vi "Mutate Status Glyph.vi"(8 "error in":errorcluster, 11 "device in":T1 format="%.0x") -> (0 "error out":errorcluster, 3 "device out":T1 format="%.0x")   [LabVIEW 2027, in "Embedded Data Logger System Explorer.lvlib"]
uses:
  Embedded Data Logger System Explorer.lvlib
  <vilib>/NI VeriStand/Custom Device API/Custom Device Item Ref.ctl
  Shared/Constants.vi
  <vilib>/NI VeriStand/Custom Device Tools/Custom Device Utility Library/NI VeriStand - Search for All Items by GUID.vi
  <vilib>/NI VeriStand/Custom Device Tools/Custom Device Utility Library/Custom Device Utility Library.lvlib
  Shared/Embedded Data Logger Shared.lvlib
  <vilib>/NI VeriStand/Custom Device API/Custom Device API.lvlib
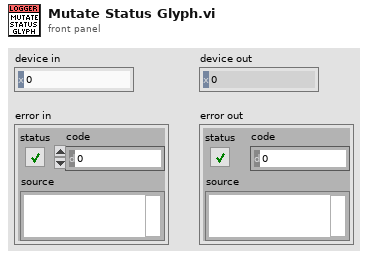
[diagram p1: front panel]
types:
  T1 = typedef "Custom Device API.lvlib/Custom Device Item Ref.ctl" = u64
  T2 = typedef "Custom Device API.lvlib/Custom Device Item Info.ctl" = cluster{"Name":string, "Is Channel":bool, "GUID":string, "Is Waveform":bool}
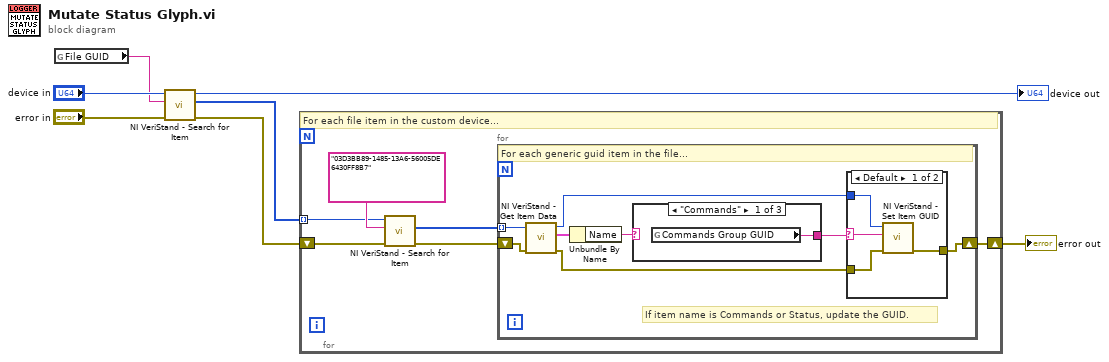
[diagram p0: block diagram]
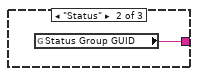
[diagram p3: hidden frame]
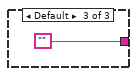
[diagram p4: hidden frame]
diagram:
  n1 = global read "Constants.vi" "File GUID"() -> (w2:string)
  n2 = call-poly <vilib>:"NI VeriStand - Search for Item.vi"("error in"="error in", "Item GUID"=w2, "Section Ref in"="device in") -> ("error out"=w6:errorcluster, "Item Refs"=w7:T1[], "Section Ref out"=→"device out":T1)  [unwired: 1 in, 5 out]
  n3 = for {
    shift-right: [w8] -> w1
    shift-left: w6 -> [w10]
    tunnel: w7 -> [w12] mode=indexing
    # "For each file item in the custom device..."
    n4 = call-poly <vilib>:"NI VeriStand - Search for Item.vi"("error in"=w10, "Item GUID"="03D3BB89-1485-13A6-56005DE6430FF8B7", "Section Ref in"=w12) -> ("error out"=w9:errorcluster, "Item Refs"=w11:T1[])  [unwired: 1 in, 6 out]
    n5 = for {
      tunnel: w11 -> [w16] mode=indexing
      shift-right: [w14] -> w8
      shift-left: w9 -> [w15]
      # "If item name is Commands or Status, update the GUID."
      # "For each generic guid item in the file..."
      n6 = call <vilib>:"NI VeriStand - Get Item Data.vi"("error in (no error)"=w15, "Item Ref in"=w16) -> ("error out"=w21:errorcluster, "Item Info"=w17:T2, "Item Ref out"=w20:T1)  [unwired: 7 out]
      n7 = Unbundle By Name(w17) -> ("Name"=w18:string)
      n8 = case shown="\"Commands\"" w18 {
        tunnel: [w27 w28 ""] -> w19
        frame "Commands" {
          n9 = global read "Constants.vi" "Commands Group GUID"() -> (w27:string)
        }
        frame "Status" {
          n10 = global read "Constants.vi" "Status Group GUID"() -> (w28:string)
        }
        frame Default {
        }
      }
      n11 = case shown="Default" w19 {
        selector: w19 -> [w24 _]
        tunnel: w20 -> [w25 _]
        tunnel: w21 -> [w23 w26]
        tunnel: [w22 w26] -> w14
        frame Default {
          n12 = call <vilib>:"NI VeriStand - Set Item GUID.vi"("error in (no error)"=w23, "GUID"=w24, "Item Ref in"=w25) -> ("error out"=w22:errorcluster)  [unwired: 7 in, 1 out]
        }
        frame "" {
        }
      }
    }
  }
  "error out" <- w1
